vi "OCUMain (D17C4V1's conflicted copy 2015-11-03).vi"() -> ()   [LabVIEW 2014]
uses:
  Command.ctl
  DataHighway.ctl
  <vilib>/ErrorRing/Error Ring.xnode
panel:
  in  "E-Stop Motors":bool
  out "DataHWay":T1
  out "ComHWay":T2 {"Speed" scale=-2.0..10.0; "Rudder" scale=-10.0..10.0}
  out "OCU Running":bool
  out "Tab Control":T3(tab)
  out "Starboard":dbl(slide) scale=20.0..60.0
  out "Front":dbl(slide) scale=20.0..60.0
  out "Boolean 5":bool
  out "Boolean 4":bool
  out "Boolean 3":bool
  out "Boolean 2":bool
  out "Boolean":bool
  in  "Beh Lights ok?":bool
  in  "myRIO ok?":bool
  in  "Prop ok?":bool
  in  "Rudder ok?":bool
  in  "Sharp IR-Lidar ok?":bool
  in  "Goto Debug?":bool
  out "MyRIO":bool
  out "Port":dbl(slide) scale=60.0..20.0
  in  "Re-Initialize":bool
  in  "Debug Robot":bool
  in  "Run Robot":bool
  in  "Stop OCU":bool
  in  "Prop Speed":dbl(knob) scale=0.05..0.1
  in  "Rudder":dbl(knob) scale=0.05..0.1
  out "Sharp IR Lidar":T4(graph)
  in  "Debug Complete?":bool
  out "RobotRunning":bool
  out "HW-Stop":bool
  in  "Exit Run":bool
  # "Press Arrow\nabove to start\nOCU running"
  # "add logic to have estop pressed when int starts"
  # "Run auto Initialize sequence.\nIndicate which functionality is ok.\nAll functions must work or choose go to debug state."
  # "Look at boat. Rudder Oscillating?"
  # "Look at boat?"
  # "Look at boat. See Red-Blue-Green?"
  # "Unit Test"
  # "Function"
  # "Press button to\nselect robot state"
  # "Robot Initialized and \nwaiting for user input"
  # "0.075 rudder center"
  # "0.075 prop off"
  # "OCU and Robot safely shut down"
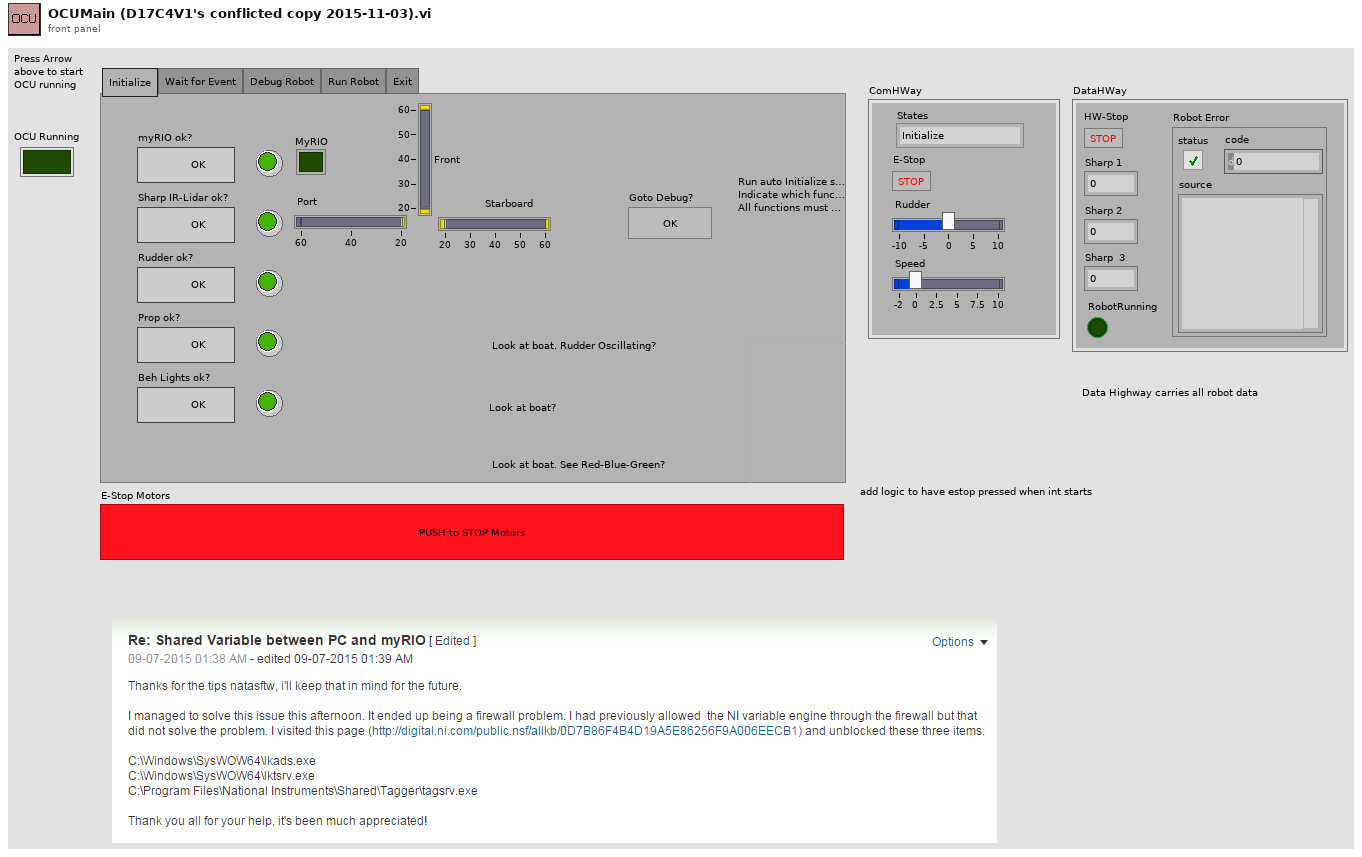
[diagram p1: front panel]
types:
  T1 = typedef "DataHighway.ctl" = cluster{"HW-Stop":bool, "Sharp 1":dbl, "Sharp 2":dbl, "Sharp  3":dbl, "RobotRunning":bool, "Robot Error":errorcluster}
  T2 = typedef "Command.ctl" = cluster{"States":enum16{"Initialize", "Wait for Event", "Debug Robot", "Run Robot", "Exit"}, "E-Stop":bool, "Rudder":dbl, "Speed":dbl}
  T3 = enum32{"Initialize", "Wait for Event", "Debug Robot", "Run Robot", "Exit"}
  T4 = cluster{"Sharp 1":dbl, "Sharp 2":dbl, "Sharp  3":dbl}
  T5 = enum16{"Initialize", "Wait for Event", "Debug Robot", "Run Robot", "Exit"}
  T6 = cluster{"Port":dbl, "Center":dbl, "Starboard":dbl}
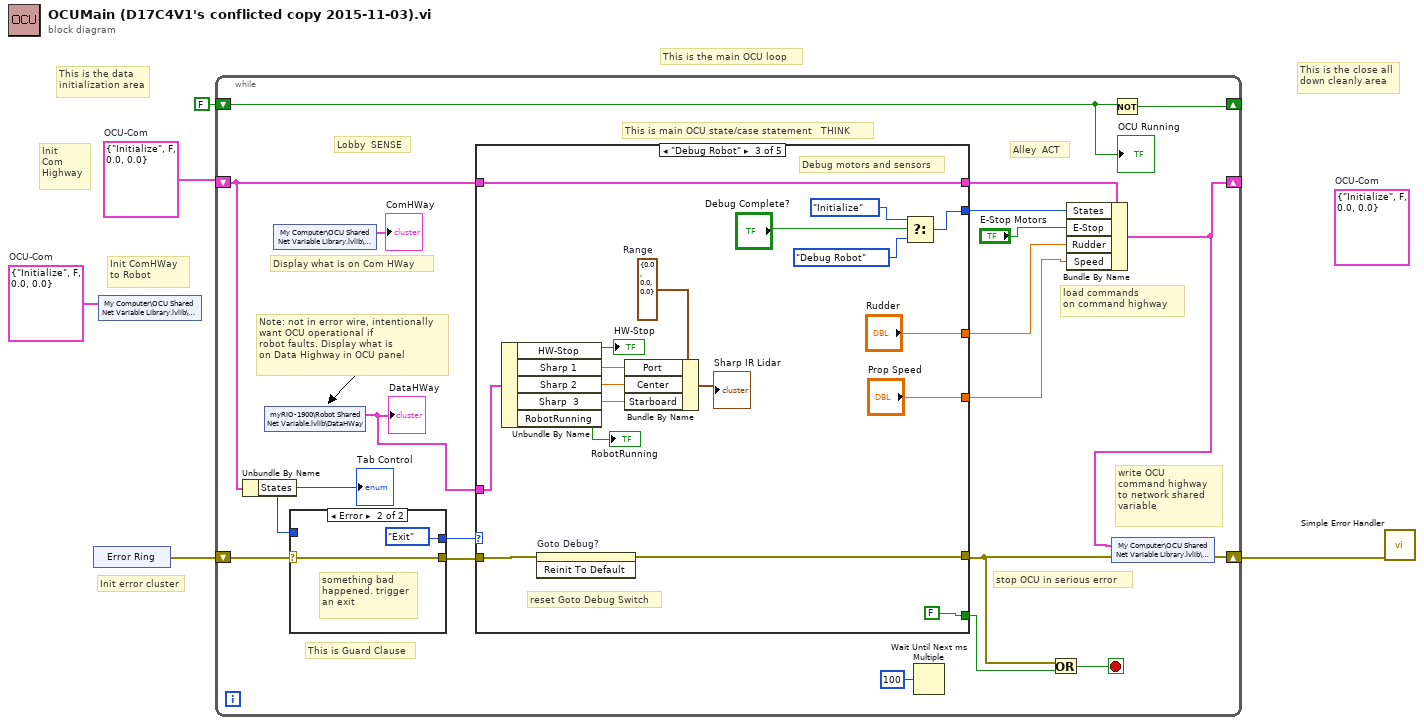
[diagram p0: block diagram]
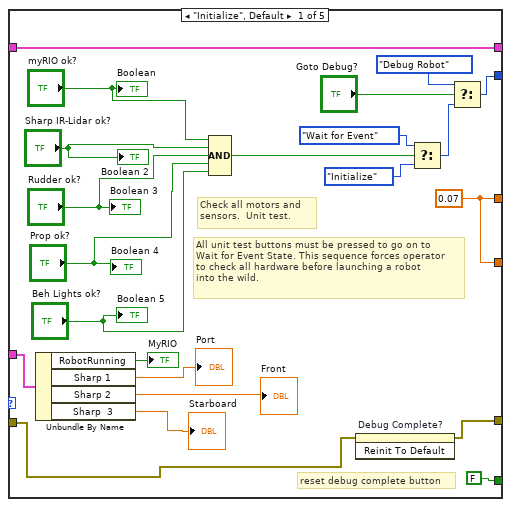
[diagram p3: hidden frame]
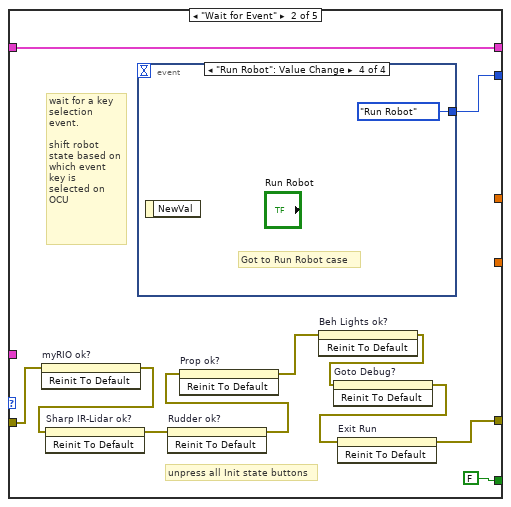
[diagram p4: hidden frame]
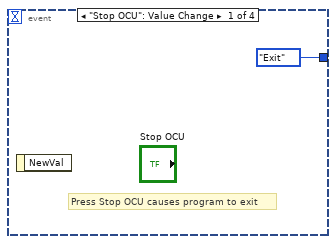
[diagram p5: hidden frame]
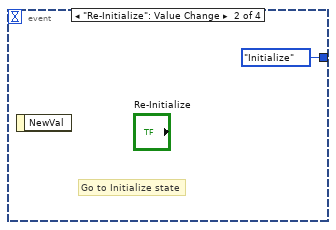
[diagram p6: hidden frame]
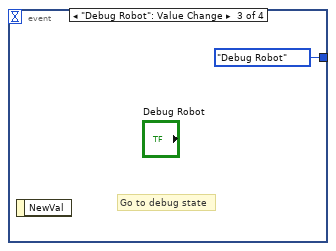
[diagram p7: hidden frame]
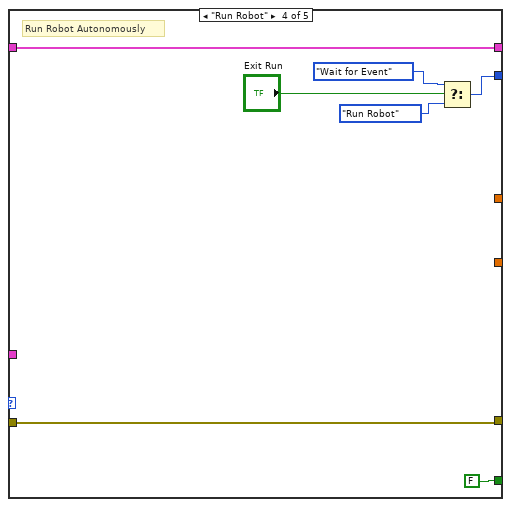
[diagram p8: hidden frame]
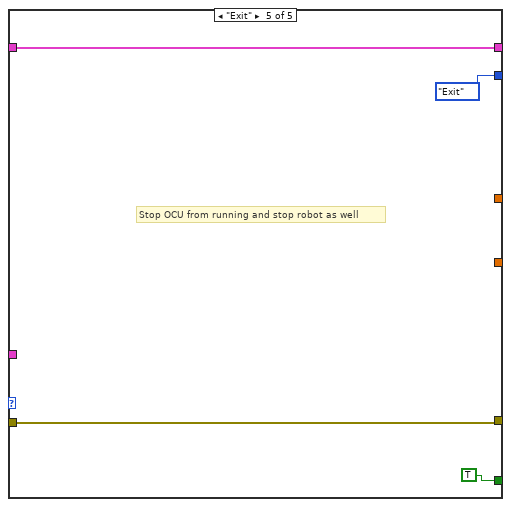
[diagram p9: hidden frame]
diagram:
  (unwired) T2 {"States"=enum."Initialize", "E-Stop"=FALSE, "Rudder"=0.0, "Speed"=0.0}  # OCU-Com
  w1 = T2 {"States"=enum."Initialize", "E-Stop"=FALSE, "Rudder"=0.0, "Speed"=0.0}  # OCU-Com
  w2 = T2 {"States"=enum."Initialize", "E-Stop"=FALSE, "Rudder"=0.0, "Speed"=0.0}  # OCU-Com
  # "Init ComHWay\nto Robot"
  # "Init error cluster"
  # "Init\nCom\nHighway"
  # "This is the close all\ndown cleanly area"
  # "This is the data\ninitialization area"
  # "This is the main OCU loop"
  n1 = xnode "Error Ring"() -> ("error out"=w4:errorcluster)
  n2 = shared-variable "My Computer\\OCU Shared Net Variable Library.lvlib\\ComHWay"(w1) -> ()  [unwired: 1 in, 1 out]
  n3 = while {
    shift-right: [w24] -> _
    shift-left: FALSE -> [w23]
    shift-right: [w13] -> w3
    shift-left: w4 -> [w22]
    shift-right: [w9] -> _
    shift-left: w2 -> [w17]
    stop <- w19 stop-if-true
    # "Note: not in error wire, intentionally\nwant OCU operational if\nrobot faults. Display what is \non Data Highway in OCU panel"
    # "load commands\non command highway"
    # "Display what is on Com HWay"
    # "write OCU  \ncommand highway\nto network shared\nvariable"
    # "stop OCU in serious error"
    # "This is Guard Clause"
    # "This is main OCU state/case statement   THINK"
    # "Alley  ACT"
    # "Lobby  SENSE"
    n4 = Unbundle By Name "Unbundle By Name"(w17) -> ("States"=w16:T5)
    "Tab Control" <- w16
    n5 = shared-variable "myRIO-1900\\Robot Shared Net Variable.lvlib\\DataHWay"() -> (w8:T1)  [unwired: 1 in, 1 out]
    "DataHWay" <- w8
    n6 = shared-variable "My Computer\\OCU Shared Net Variable Library.lvlib\\ComHWay"() -> (→"ComHWay":T2)  [unwired: 1 in, 1 out]
    n7 = case shown="Error" w22 {
      selector: w22 -> [w27 w29]
      tunnel: [w27 w29] -> w21
      tunnel: w16 -> [w26 _]
      tunnel: [w26 T5."Exit" ("States")] -> w18
      frame No Error {
      }
      frame Error {
        # "something bad\nhappened. trigger\nan exit"
      }
    }
    n8 = case shown="\"Debug Robot\"" w18 {
      tunnel: [w50 w61 w82 w89 T5."Exit" ("States")] -> w15
      tunnel: [FALSE FALSE FALSE FALSE TRUE] -> w20
      tunnel: w21 -> [w35 w60 w79 w87 w93]
      tunnel: [w38 w52 w78 w87 w93] -> w14
      tunnel: w17 -> [w37 w54 w77 w85 w92]
      tunnel: [w37 w54 w77 w85 w92] -> w12
      tunnel: w8 -> [w36 _ w76 _ _]
      tunnel: [w30 _ "Rudder" _ _] -> w7
      tunnel: [w30 _ "Prop Speed" _ _] -> w6
      frame "Initialize", Default {
        w30 = 0.07 ("Rudder")
        # "reset debug complete button"
        # "All unit test buttons must be pressed to go on to \nWait for Event State. This sequence forces operator\nto check all hardware before launching a robot\ninto the wild."
        # "Check all motors and \nsensors.  Unit test."
        n9 = Unbundle By Name(w36) -> ("RobotRunning"=→"MyRIO":bool, "Sharp 1"=→"Port":dbl, "Sharp 2"=→"Front":dbl, "Sharp  3"=→"Starboard":dbl)
        n10 = Compound Arithmetic op=AND("myRIO ok?", "Sharp IR-Lidar ok?", "Rudder ok?", "Prop ok?", "Beh Lights ok?") -> (w39:bool)
        n11 = invoke on="Debug Complete?" class="Bool (strict)" method="Reinit To Default"(error in=w35) -> (error out=w38:errorcluster)  [unwired: 2 in, 2 out]
        n12 = Select ("Select next state")(t=T5."Wait for Event" ("States"), s=w39, f=T5."Initialize") -> (s? t:f=w47:T5)
        n13 = Select ("Select next state")(t=T5."Debug Robot" ("f"), s="Goto Debug?", f=w47) -> (s? t:f=w50:T5)
        "Boolean" <- "myRIO ok?"
        "Boolean 2" <- "Sharp IR-Lidar ok?"
        "Boolean 3" <- "Rudder ok?"
        "Boolean 4" <- "Prop ok?"
        "Boolean 5" <- "Beh Lights ok?"
      }
      frame "Wait for Event" {
        # "unpress all Init state buttons"
        # "wait for a key \nselection\nevent.\n\nshift robot\nstate based on\nwhich event\nkey is\nselected on \nOCU"
        n14 = invoke on="myRIO ok?" class="Bool (strict)" method="Reinit To Default"(error in=w60) -> (error out=w59:errorcluster)  [unwired: 2 in, 2 out]
        n15 = invoke on="Sharp IR-Lidar ok?" class="Bool (strict)" method="Reinit To Default"(error in=w59) -> (error out=w58:errorcluster)  [unwired: 2 in, 2 out]
        n16 = event shown="[3] \"Run Robot\": Value Change" {
          selector: _ -> [_ _ _ _]
          dyn-events: _ -> [_ _ _ _]
          timeout: _ -> [_ _ _ _]
          tunnel: [T5."Exit" ("States") T5."Initialize" ("States") T5."Debug Robot" ("States") T5."Run Robot" ("States")] -> w61
          event "Stop OCU": Value Change {
            # "Press Stop OCU causes program to exit"
            n17 = event-data() -> ()  [unwired: 1 in, 1 out]
          }
          event "Re-Initialize": Value Change {
            # "Go to Initialize state"
            n18 = event-data() -> ()  [unwired: 1 in, 1 out]
          }
          event "Debug Robot": Value Change {
            # "Go to debug state"
            n19 = event-data() -> ()  [unwired: 1 in, 1 out]
          }
          event "Run Robot": Value Change {
            # "Got to Run Robot case"
            n20 = event-data() -> ()  [unwired: 1 in, 1 out]
          }
        }
        n21 = invoke on="Rudder ok?" class="Bool (strict)" method="Reinit To Default"(error in=w58) -> (error out=w57:errorcluster)  [unwired: 2 in, 2 out]
        n22 = invoke on="Prop ok?" class="Bool (strict)" method="Reinit To Default"(error in=w57) -> (error out=w56:errorcluster)  [unwired: 2 in, 2 out]
        n23 = invoke on="Beh Lights ok?" class="Bool (strict)" method="Reinit To Default"(error in=w56) -> (error out=w55:errorcluster)  [unwired: 2 in, 2 out]
        n24 = invoke on="Goto Debug?" class="Bool (strict)" method="Reinit To Default"(error in=w55) -> (error out=w53:errorcluster)  [unwired: 2 in, 2 out]
        n25 = invoke on="Exit Run" class="Bool (strict)" method="Reinit To Default"(error in=w53) -> (error out=w52:errorcluster)  [unwired: 2 in, 2 out]
      }
      frame "Debug Robot" {
        w70 = T6 {"Port"=0.0, "Center"=0.0, "Starboard"=0.0}  # Range
        # "reset Goto Debug Switch"
        # "Debug motors and sensors"
        n26 = Unbundle By Name "Unbundle By Name"(w76) -> ("HW-Stop"=→"HW-Stop":bool, "Sharp 1"=w73:dbl, "Sharp 2"=w72:dbl, "Sharp  3"=w71:dbl, "RobotRunning"=→"RobotRunning":bool)
        n27 = invoke on="Goto Debug?" class="Bool (strict)" method="Reinit To Default"(error in=w79) -> (error out=w78:errorcluster)  [unwired: 2 in, 2 out]
        n28 = Bundle By Name(cluster=w70, "Port"=w73, "Center"=w72, "Starboard"=w71) -> (→"Sharp IR Lidar":T6)
        n29 = Select(t=T5."Initialize" ("States"), s="Debug Complete?", f=T5."Debug Robot") -> (s? t:f=w82:T5)
      }
      frame "Run Robot" {
        # "Run Robot Autonomously"
        n30 = Select(t=T5."Wait for Event" ("States"), s="Exit Run", f=T5."Run Robot") -> (s? t:f=w89:T5)
      }
      frame "Exit" {
        # "Stop OCU from running and stop robot as well"
      }
    }
    n31 = Wait Until Next ms Multiple(millisecond multiple=u32 100) -> ()  [unwired: 1 out]
    n32 = Or(x=w14, y=w20) -> (x .or. y?=w19:bool)
    n33 = Bundle By Name(cluster=w12, "States"=w15, "E-Stop"="E-Stop Motors", "Rudder"=w7, "Speed"=w6) -> (w9:T2)
    n34 = Not(x=w23) -> (.not. x?=w24:bool)
    n35 = shared-variable "My Computer\\OCU Shared Net Variable Library.lvlib\\ComHWay"(w9, error in=w14) -> (error out=w13:errorcluster)
    "OCU Running" <- w23
  }
  n36 = call <vilib>:"Simple Error Handler.vi"("error in (no error)"=w3) -> ()  [unwired: 4 in, 5 out]
